vi "Read All.vi"(8 "Error In":errorcluster) -> (0 "Error Out":errorcluster)   [LabVIEW 2018, in "Tests.lvlib" / "Readers.lvlib" / "String.lvlib"]
uses:
  String.lvlib
  src/Toolkit/Public/Readers/Public/String/String.lvclass
  <vilib>/addons/_JKI Toolkits/Caraya/classes/Test/Test.lvclass
  <vilib>/addons/_JKI Toolkits/Caraya/classes/Assert/Assert.lvclass
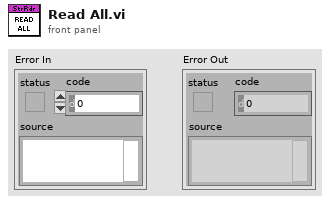
[diagram p1: front panel]
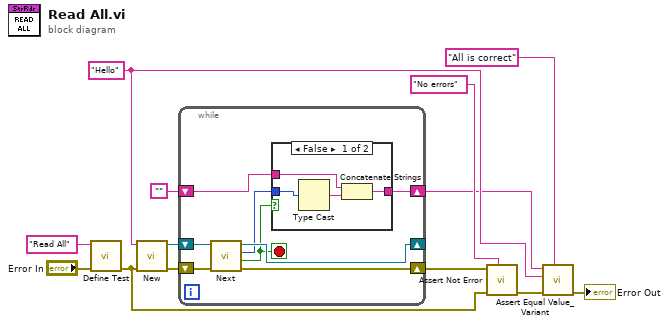
[diagram p0: block diagram]
diagram:
  w3 = "Hello" ("String")
  n1 = call <vilib>:"Define Test.vi"("error in (no error)"="Error In", "Label (VI Title)"="Read All") -> ("error out"=w8:errorcluster)  [unwired: 9 in]
  n2 = call "New.vi"("Error In"=w8, "String"=w3) -> ("Error Out"=w10:errorcluster, "String"=w11:refnum<class "String.lvclass">)  [unwired: 8 in]
  n3 = while {
    shift-right: [w19] -> w9
    shift-left: w10 -> [w20]
    shift-right: [w18] -> _
    shift-left: w11 -> [w21]
    shift-right: [w15] -> w1
    shift-left: "" -> [w16]
    stop <- w17 stop-if-true
    n4 = call-dynamic "Next.vi"("Error In"=w20, "Reader In"=w21) -> ("Error Out"=w19:errorcluster, "Done"=w17:bool, "Character"=w14:u8, "Reader Out"=w18:refnum<class "String.lvclass">)  [unwired: 6 in]
    n5 = case shown="False" w17 {
      tunnel: w16 -> [w25 w26]
      tunnel: [w24 w26] -> w15
      tunnel: w14 -> [w23 _]
      frame False {
        n6 = Type Cast(x=w23) -> (*(type *) &x=w22:string)  [unwired: 1 in]
        n7 = Concatenate Strings(w25, w22) -> (w24:string)
      }
      frame True {
      }
    }
  }
  n8 = call <vilib>:"Assert Not Error.vi"("Label"="No errors", "error in (no error)"=w8, "Not Error?"=w9) -> ("error out"=w6:errorcluster)  [unwired: 8 in]
  n9 = call <vilib>:"Assert Equal Value_Variant.vi"("Label"="All is correct", "error in (no error)"=w6, "Y"=w3, "X"=w1) -> ("error out"=→"Error Out":errorcluster)  [unwired: 7 in]
